vi "Test View Broadcast When View is Shown.vi"(8 "error in (no error)":errorcluster, 11 "UI View Test In":refnum<class "View Dev Test.lvclass">) -> (0 "error out":errorcluster, 3 "UI View Test Out":refnum<class "View Dev Test.lvclass">)   [LabVIEW 2020, in "View Dev Test.lvclass"]
uses:
  View Dev Test.lvclass
  C:/Program Files (x86)/National Instruments/LabVIEW 2020/vi.lib/Astemes/LUnit/Test Case.lvclass
  source/Framework/Process/Process.lvclass/Process.ctl
  source/Framework/View/View.lvclass/View.ctl
  <vilib>/Astemes/LUnit/Test Case.lvclass/Test Case.ctl
  <vilib>/Astemes/LUnit/LUnit Assertion Result.lvclass/LUnit Assertion Result.ctl
  <vilib>/Astemes/LUnit/LUnit Test Case Result.lvclass/LUnit Test Case Result.ctl
  <vilib>/Astemes/LUnit/LUnit Method Result.lvclass/LUnit Method Result.ctl
  c28a26a2-0c44-4f32-8aa2-12100485784b.vi
  source/Framework/Process/Public/Lifecycle/Get Lifecycle State.vi
  source/Framework/Process/Protected/Messaging/Enqueue Message.vi
  source/Framework/View/Public/Get View VI Reference.vi
  source/Framework/Broadcast Event Helpers/Execution timer.vi
  source/Framework/Process/Private/SubVIs/Wait for finish.vi
  source/Framework/Process/Private/SubVIs/Set Lifecycle State.vi
  <vilib>/Astemes/LUnit/Palette/Pass.vi
  <vilib>/Astemes/LUnit/Palette/Fail.vi
  <vilib>/Astemes/LUnit/Compare Variants.vi
  <vilib>/Astemes/LUnit/Describe Comparison.vi
  <vilib>/Astemes/LUnit/Set Assertion Type.vi
  <vilib>/Utility/error.llb/Clear Errors.vi
  source/Framework/Process/Private/SubVIs/Handle Debug Data.vi
  source/Framework/Process/Protected/Messaging/Request Message.vi
  <vilib>/Astemes/LUnit/Add test result.vi
  <vilib>/Astemes/LUnit/LUnit Write Passed.vi
  <vilib>/Astemes/LUnit/LUnit Write Message.vi
  <vilib>/Astemes/LUnit/LUnit Write Description.vi
  <vilib>/Astemes/LUnit/Variant to string.vi
  <vilib>/Astemes/LUnit/LUnit Write Assertion Type.vi
  source/Framework/Logging/Log Debug.vi
  <vilib>/AdvancedString/1D String Array to Delimited String.vi
  <vilib>/Utility/High Resolution Relative Seconds.vi
  source/Framework/Process/Private/SubVIs/Enqueue Request Message.vi
  <vilib>/Astemes/LUnit/LUnit Record Assertion Result.vi
  <vilib>/Astemes/LUnit/LUnit Aggregate Assertion Results.vi
  <vilib>/Astemes/LUnit/Assertion Result/LUnit Read Status.vi
  <vilib>/Astemes/LUnit/LUnit Read Message.vi
  <vilib>/Astemes/LUnit/LUnit Read Description.vi
  <vilib>/Astemes/LUnit/Method Result/LUnit Merge Status.vi
  <vilib>/Astemes/LUnit/LUnit Concatenate result strings.vi
  source/Framework/View/View.lvclass
  C:/Git/astemes-triarc-framework/source/Framework/Process/Process.lvclass
  <vilib>/Utility/error.llb/Error Cluster From Error Code.vi
  source/Framework/Process/Public/Read Name.vi
  source/Framework/Process/Private/SubVIs/Wait for Response Message.vi
  source/Framework/Broadcast Event Helpers/Dequeue Broadcast Message.vi
  <vilib>/Utility/Data Type/Get Type Information.vi
  <vilib>/Utility/LVClass/Get LV Class Name.vi
  <vilib>/Astemes/LUnit/LUnit Assertion Result.lvclass
  source/Framework/Process/Process.lvclass
  source/Framework/Broadcast Event Helpers/Broadcast Event Helpers.lvlib
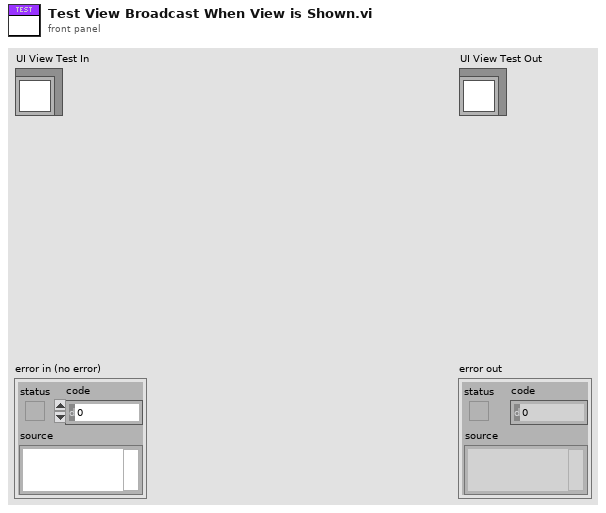
[diagram p1: front panel]
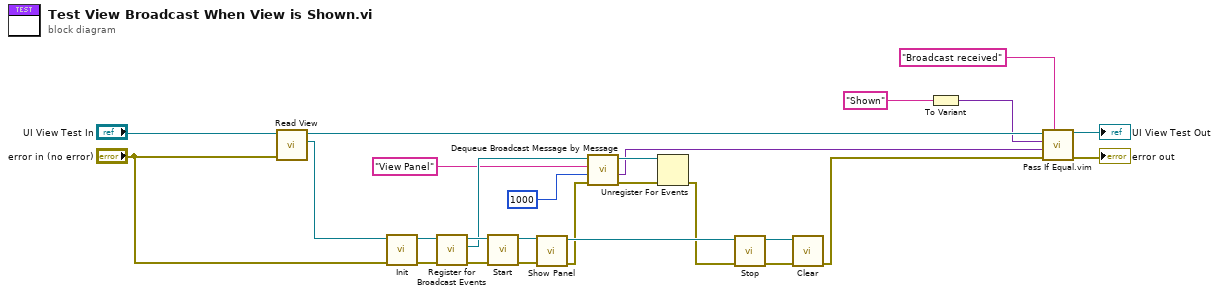
[diagram p0: block diagram]
diagram:
  n1 = call "Read View.vi"("error in (no error)"="error in (no error)", "View Test In"="UI View Test In") -> ("View"=w22:refnum<class "View.lvclass">, "View Test Out"=w25:refnum<class "View Dev Test.lvclass">)  [unwired: 7 in, 1 out]
  n2 = call-dynamic "Init.vi"("error in (no error)"="error in (no error)", "View In"=w22) -> ("error out"=w17:errorcluster, "View Out"=w13:refnum<class "View.lvclass">)  [unwired: 8 in]
  n3 = call "Register for Broadcast Events.vi"("error in (no error)"=w17, "Process In"=w13) -> ("error out"=w14:errorcluster, "Event Registration Refnum Out"=w11:refnum<event-registration>, "Process Out"=w12:refnum<class "View.lvclass">)  [unwired: 7 in]
  n4 = call "Start.vi"("error in (no error)"=w14, "Process In"=w12) -> ("error out"=w20:errorcluster, "Process Out"=w21:refnum<class "View.lvclass">)  [unwired: 7 in, 1 out]
  n5 = call "Show Panel.vi"("error in (no error)"=w20, "View In"=w21) -> ("error out"=w2:errorcluster, "View Out"=w15:refnum<class "View.lvclass">)  [unwired: 8 in]
  n6 = call "Dequeue Broadcast Message by Message.vi"("error in (no error)"=w2, "Timeout (-1)"=1000, "Message"="View Panel", "Event Registration Refnum"=w11) -> ("error out"=w3:errorcluster, "Message Data"=w6:variant, "Event Registration Refnum Out"=w8:refnum<event-registration>)  [unwired: 3 in, 2 out]
  n7 = Unregister For Events(event registration refnum=w8, error in=w3) -> (error out=w1:errorcluster)
  n8 = call "Stop.vi"("error in (no error)"=w1, "Process In"=w15) -> ("error out"=w18:errorcluster, "Process Out"=w19:refnum<class "View.lvclass">)  [unwired: 7 in, 1 out]
  n9 = call-dynamic "Clear.vi"("error in (no error)"=w18, "View In"=w19) -> ("error out"=w7:errorcluster)  [unwired: 9 in]
  n10 = To Variant(anything="Shown") -> (Variant=w4:variant)
  n11 = call "Pass If Equal.vim"("Description"="Broadcast received", "error in (no error)"=w7, "Actual"=w6, "Expected"=w4, "LUnit Test Case In"=w25) -> ("error out"=→"error out":errorcluster, "LUnit Test Case Out"=→"UI View Test Out":refnum<class "View Dev Test.lvclass">)  [unwired: 5 in]
